vi "Init Variables.vi"(8 "error in (no error)":errorcluster) -> (0 "error out":errorcluster)   [LabVIEW 2016]
uses:
  Controls/Operational Modes.ctl
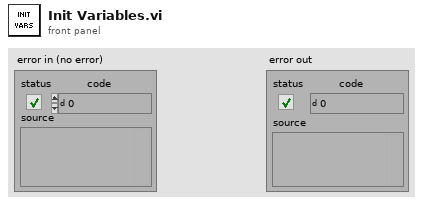
[diagram p1: front panel]
types:
  T1 = typedef "Operational Modes.ctl" = enum16{"Sci", "Sci-LFC", "Solar", "Solar-LFC", "LFC", "LFC-Sim", "LFC-Both", "ThAr", "ThAr-LFC", "Flat", "ExtFlat", "ExtFlat-Sim", "ExtFlat-Both", "Qtz", "ExtQtz", "ExtQtz-Sim", "ExtQtz-Both", "Dark", "Manual", "Off"}
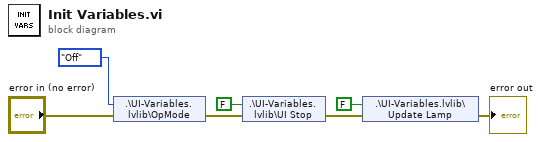
[diagram p0: block diagram]
diagram:
  n1 = shared-variable ".\\UI-Variables.lvlib\\OpMode"(Operational_Modes."Off" ("OpMode"), error in="error in (no error)") -> (error out=w6:errorcluster)
  n2 = shared-variable ".\\UI-Variables.lvlib\\UI Stop"(FALSE ("UI Stop"), error in=w6) -> (error out=w7:errorcluster)
  n3 = shared-variable ".\\UI-Variables.lvlib\\Update Lamp"(FALSE ("Update Lamp"), error in=w7) -> (error out=→"error out":errorcluster)
